vi "Camera.vi"() -> ()   [LabVIEW 2016]
uses:
  <vilib>/rvi/Emulation/niFpgaGetClockAttributes.vi
  <vilib>/rvi/Emulation/niFpgaSctlEmulationGetInTimedLoop.vi
  <vilib>/rvi/Emulation/niFpgaEmulationReportErrorSimple.vi
  <vilib>/rvi/eio/common/nirviEmuTemplateMethod_errors.vi
  <vilib>/rvi/Emulation/niFpgaCriticalErrorInLSC.vi
  <vilib>/eio/EIONode/EIONode.xnode
panel:
  in  "Fluorenscen Camera = R(100Hz = 200, 50Hz = 400)":i16=200
  in  "Tlow = t":i16=9
  in  "Fly View Frame Rate = R":i16=10
  in  "Arena View Frame Rate = R":i16=100
  out "Camera flash time":i16
  in  "Camera flash time t":i16
  in  "Flash":bool
  # "** Frequency  = 1 / (Fly View R * 0.0001)   i.e R = 10, Frequency = 1000Hz"
  # "**T period = R*100µs,      T low = t*100 µs"
  # "** Frequency  = 1 / (R * 0.0001)   i.e R = 100, Frequency = 100Hz"
  # "** Trigger the fluorenscence camera (Arena View R - x ) *100 microseconds earlier\n      i.e Arena View R = 100, x = 98,\n           offset x = (100 - 98) * 100 µs = 200 µs"
  # "** Camera flash time is set to be the time for triggering the flash at the end of every video.\n** The unit is second."
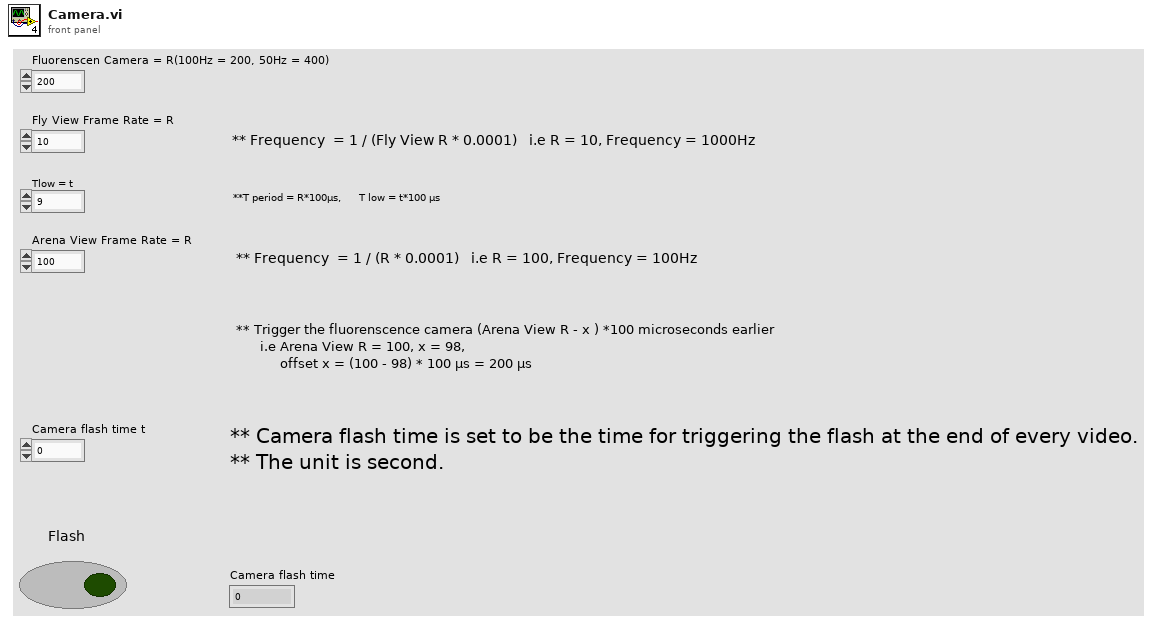
[diagram p1: front panel]
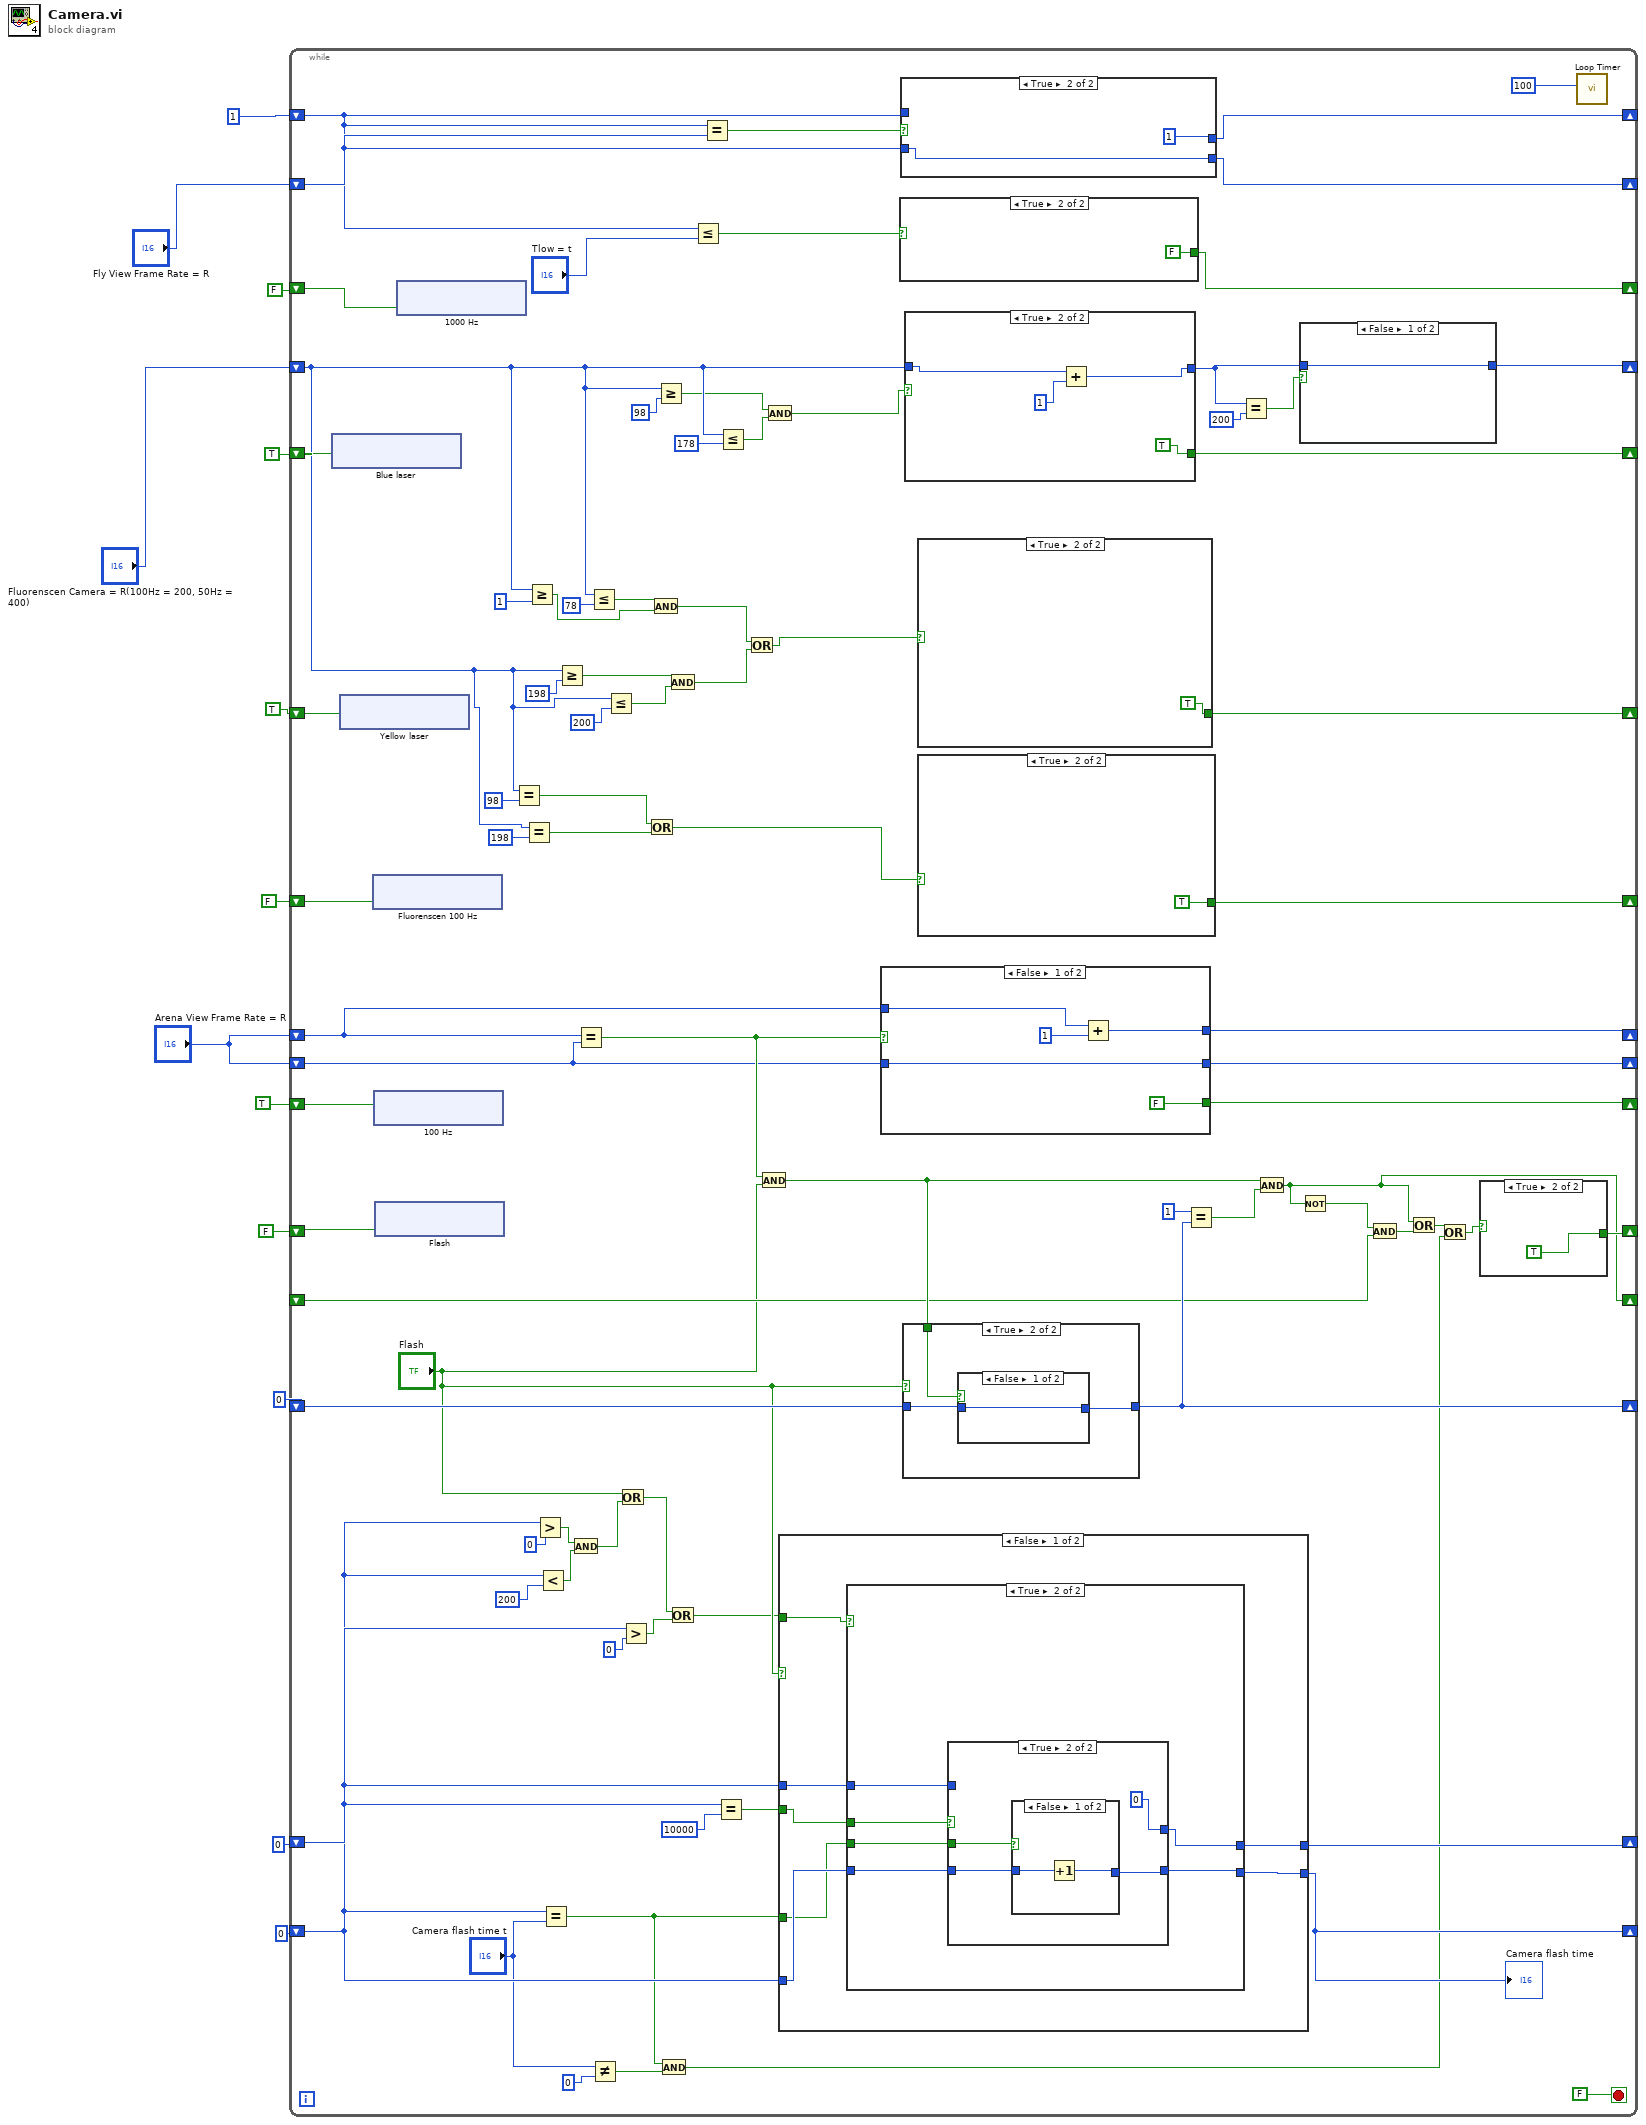
[diagram p0: block diagram]
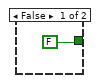
[diagram p2: hidden frame]
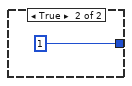
[diagram p3: hidden frame]
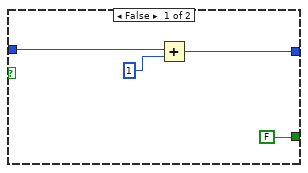
[diagram p4: hidden frame]
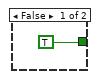
[diagram p5: hidden frame]
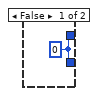
[diagram p6: hidden frame]
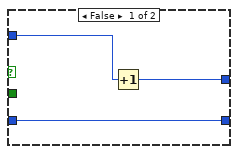
[diagram p7: hidden frame]
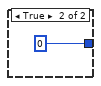
[diagram p8: hidden frame]
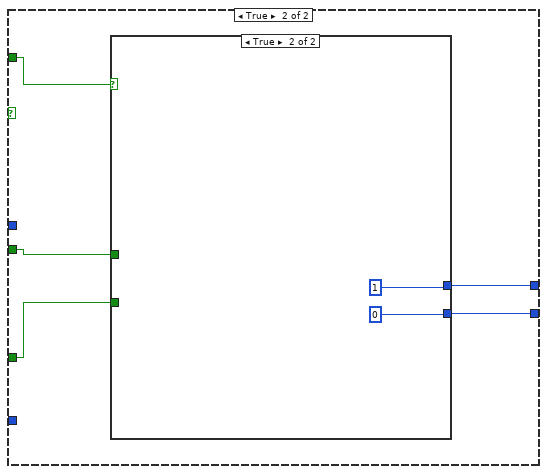
[diagram p9: hidden frame]
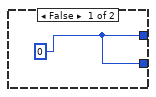
[diagram p10: hidden frame]
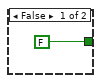
[diagram p11: hidden frame]
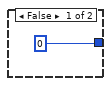
[diagram p12: hidden frame]
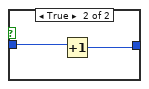
[diagram p13: hidden frame]
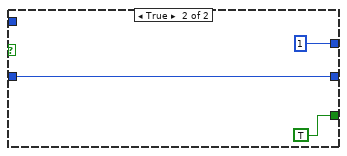
[diagram p14: hidden frame]
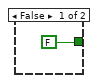
[diagram p15: hidden frame]
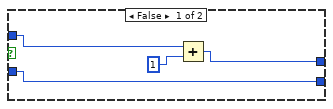
[diagram p16: hidden frame]
diagram:
  n1 = while {
    shift-right: [w48] -> _
    shift-left: FALSE -> [w97]
    shift-right: [w95] -> _
    shift-left: i16 1 -> [w44]
    shift-right: [w93] -> _
    shift-left: FALSE -> [w94]
    shift-right: [w92] -> _
    shift-left: TRUE -> [w87]
    shift-right: [w91] -> _
    shift-left: "Arena View Frame Rate = R" -> [w82]
    shift-right: [w84] -> _
    shift-left: i16 0 -> [w88]
    shift-right: [w80] -> _
    shift-left: FALSE -> [w81]
    shift-right: [w76] -> _
    shift-left: _ -> [w77]
    shift-right: [w70] -> _
    shift-left: i16 0 -> [w63]
    shift-right: [w71] -> _
    shift-left: i16 0 -> [w57]
    shift-right: [w51] -> _
    shift-left: "Arena View Frame Rate = R" -> [w50]
    shift-right: [w49] -> _
    shift-left: "Fly View Frame Rate = R" -> [w47]
    shift-right: [w39] -> _
    shift-left: "Fluorenscen Camera = R(100Hz = 200, 50Hz = 400)" -> [w17]
    shift-right: [w42] -> _
    shift-left: TRUE -> [w43]
    shift-right: [w36] -> _
    shift-left: TRUE -> [w37]
    stop <- FALSE stop-if-true
    n2 = xnode "Blue laser"("ConnectorC/DIO4"=w43) -> ()  [unwired: 1 in, 1 out]
    n3 = xnode "Yellow laser"("ConnectorC/DIO5"=w37) -> ()  [unwired: 1 in, 1 out]
    n4 = xnode "Fluorenscen 100 Hz"("ConnectorC/DIO1"=w94) -> ()  [unwired: 1 in, 1 out]
    n5 = xnode "100 Hz"("ConnectorC/DIO2"=w87) -> ()  [unwired: 1 in, 1 out]
    n6 = xnode "Flash"("ConnectorC/DIO3"=w81) -> ()  [unwired: 1 in, 1 out]
    n7 = xnode "1000 Hz"("ConnectorC/DIO0"=w97) -> ()  [unwired: 1 in, 1 out]
    n8 = Equal?(x=w17, y=i16 98) -> (x = y?=w34:bool)
    n9 = Equal?(x=w17, y=i16 198) -> (x = y?=w32:bool)
    n10 = Greater Or Equal?(x=w17, y=i16 1) -> (x >= y?=w21:bool)
    n11 = Greater?(x=w57, y=i16 0) -> (0:w60:bool)
    n12 = Less?(x=w57, y=i16 200) -> (x < y?=w59:bool)
    n13 = Equal?(x=w57, y="Camera flash time t") -> (x = y?=w53:bool)
    n14 = Greater Or Equal?(x=w17, y=i16 198) -> (x >= y?=w24:bool)
    n15 = And(x=w60, y=w59) -> (x .and. y?=w58:bool)
    n16 = Equal?(x=w82, y=w50) -> (x = y?=w89:bool)
    n17 = Less Or Equal?(x=w17, y=i16 78) -> (x <= y?=w22:bool)
    n18 = Not Equal?(x="Camera flash time t", y=i16 0) -> (x != y?=w54:bool)
    n19 = Less Or Equal?(x=w17, y=i16 200) -> (x <= y?=w25:bool)
    n20 = Or(x="Flash", y=w58) -> (x .or. y?=w65:bool)
    n21 = Greater?(x=w63, y=i16 0) -> (0:w66:bool)
    n22 = Or(x=w34, y=w32) -> (x .or. y?=w31:bool)
    n23 = And(x=w22, y=w21) -> (x .and. y?=w20:bool)
    n24 = Greater Or Equal?(x=w17, y=i16 98) -> (x >= y?=w16:bool)
    n25 = And(x=w53, y=w54) -> (x .and. y?=w52:bool)
    n26 = And(x=w24, y=w25) -> (x .and. y?=w23:bool)
    n27 = Or(x=w65, y=w66) -> (x .or. y?=w64:bool)
    n28 = Less Or Equal?(x=w44, y="Tlow = t") -> (x <= y?=w46:bool)
    n29 = Equal?(x=w44, y=w47) -> (x = y?=w90:bool)
    n30 = Equal?(x=w63, y=i16 10000) -> (x = y?=w69:bool)
    n31 = Less Or Equal?(x=w17, y=i16 178) -> (x <= y?=w15:bool)
    n32 = Or(x=w20, y=w23) -> (x .or. y?=w30:bool)
    n33 = And(x=w89, y="Flash") -> (x .and. y?=w86:bool)
    n34 = And(x=w16, y=w15) -> (x .and. y?=w14:bool)
    n35 = case shown="False" "Flash" {
      tunnel: [w117 w140] -> w71
      tunnel: [w118 w139] -> w70
      tunnel: w63 -> [w115 _]
      tunnel: w69 -> [w116 w138]
      tunnel: w53 -> [w112 w137]
      tunnel: w57 -> [w114 _]
      tunnel: w64 -> [w113 w136]
      frame False {
        n36 = case shown="True" w113 {
          tunnel: [w119 w123] -> w118
          tunnel: [w119 w122] -> w117
          tunnel: w116 -> [_ w125]
          tunnel: w115 -> [_ w124]
          tunnel: w114 -> [_ w121]
          tunnel: w112 -> [_ w120]
          frame False {
            w119 = i16 0
          }
          frame True {
            n37 = case shown="True" w125 {
              tunnel: w124 -> [w128 _]
              tunnel: [w127 i16 0] -> w123
              tunnel: [w126 w131] -> w122
              tunnel: w121 -> [w126 w130]
              tunnel: w120 -> [_ w129]
              frame False {
                n38 = Increment(x=w128) -> (x+1=w127:i16)
              }
              frame True {
                n39 = case shown="False" w129 {
                  tunnel: [w133 i16 0] -> w131
                  tunnel: w130 -> [w134 _]
                  frame False {
                    n40 = Increment(x=w134) -> (x+1=w133:i16)
                  }
                  frame True {
                  }
                }
              }
            }
          }
        }
      }
      frame True {
        n41 = case shown="True" w136 {
          tunnel: [w141 i16 1] -> w139
          tunnel: w137 -> [_ _]
          tunnel: [w141 i16 0] -> w140
          tunnel: w138 -> [_ _]
          frame False {
            w141 = i16 0
          }
          frame True {
          }
        }
      }
    }
    "Camera flash time" <- w71
    n42 = case shown="False" w89 {
      tunnel: [FALSE TRUE] -> w92
      tunnel: [w155 i16 1] -> w91
      tunnel: w82 -> [w157 _]
      tunnel: [w153 w158] -> w51
      tunnel: w50 -> [w153 w158]
      frame False {
        n43 = Add(x=w157, y=i16 1) -> (x+y=w155:i16)
      }
      frame True {
      }
    }
    n44 = case shown="True" w46 {
      tunnel: [TRUE FALSE] -> w48
      frame False {
      }
      frame True {
      }
    }
    n45 = case shown="True" w90 {
      tunnel: [w165 i16 1] -> w95
      tunnel: w44 -> [w164 _]
      tunnel: [w163 w167] -> w49
      tunnel: w47 -> [w163 w167]
      frame False {
        n46 = Add(x=w164, y=i16 1) -> (x+y=w165:i16)
      }
      frame True {
      }
    }
    n47 = case shown="True" "Flash" {
      tunnel: w88 -> [_ w148]
      tunnel: [i16 0 w147] -> w84
      tunnel: w86 -> [_ w149]
      frame False {
      }
      frame True {
        n48 = case shown="False" w149 {
          tunnel: w148 -> [w150 w152]
          tunnel: [w150 w151] -> w147
          frame False {
          }
          frame True {
            n49 = Increment(x=w152) -> (x+1=w151:i16)
          }
        }
      }
    }
    n50 = case shown="True" w14 {
      tunnel: w17 -> [w104 w107]
      tunnel: [w103 w106] -> w38
      tunnel: [FALSE TRUE] -> w42
      frame False {
        n51 = Add(x=w104, y=i16 1) -> (x+y=w103:i16)
      }
      frame True {
        n52 = Add(x=w107, y=i16 1) -> (x+y=w106:i16)
      }
    }
    n53 = case shown="True" w30 {
      tunnel: [FALSE TRUE] -> w36
      frame False {
      }
      frame True {
      }
    }
    n54 = case shown="True" w31 {
      tunnel: [FALSE TRUE] -> w93
      frame False {
      }
      frame True {
      }
    }
    n55 = Equal?(x=i16 1, y=w84) -> (x = y?=w83:bool)
    n56 = Equal?(x=w38, y=i16 200) -> (x = y?=w40:bool)
    n57 = And(x=w86, y=w83) -> (x .and. y?=w76:bool)
    n58 = case shown="False" w40 {
      tunnel: [w100 i16 1] -> w39
      tunnel: w38 -> [w100 _]
      frame False {
      }
      frame True {
      }
    }
    n59 = Not(x=w76) -> (.not. x?=w78:bool)
    n60 = And(x=w78, y=w77) -> (x .and. y?=w79:bool)
    n61 = Or(x=w76, y=w79) -> (x .or. y?=w74:bool)
    n62 = Or(x=w74, y=w52) -> (x .or. y?=w73:bool)
    n63 = case shown="True" w73 {
      tunnel: [FALSE TRUE] -> w80
      frame False {
      }
      frame True {
      }
    }
    n64 = call "Loop Timer"("Count(uSec)"=u32 100) -> ()  [unwired: 1 out]
  }
